vi "S7NetCom Simple Reply Decoder.vi"(11 "Live data":T1[](array[typedef])=[50, 3, 0, 0, 4, 47, 0, 2, 0, 5, 0, 0, 4, 1, 255, 4, 0, 8, 49] format="0x%02x") -> ()   [LabVIEW 2014]
doc: "____\nCopyright (c) 2019 Hampel Software Engineering (HSE), released under BSD license. More info can be found on https://dokuwiki.hampel-soft.com/code/hse/s7netcom. Original code published by Marc Christenson, Sisu Devices."
uses:
  Controls/S7NetCom_HexByte.ctl
  S7NetCom.lvclass
panel:
  out "Error":u8[](array[numeric]) format="%02x"
  out "Tab Control":enum32{"CR", "DT"}(tab)
  out "Params & Data":u8[](array[numeric]) format="%.0x"
  out "Header":u8[](array[numeric]) format="%02x"
  # "0x32\tProtocol ID"
  # "0x01 (request), 0x02 (acknowledge), 0x03 (re- sponse), \n0x07 (request user data), or 0x08 (request server control)"
  # "0x00\tReserved"
  # "0x00\tReserved"
  # "[4-5]\t\tPDU Reference (user defineable)"
  # "[6-7]\t\tParameter Length"
  # "[8-9]\t\tData Length"
  # "original message"
  # "Max AmQ (parallel jobs with ack) calling"
  # "Max AmQ (parallel jobs with ack) called"
  # "Actual PDU Length"
  # "Function code (F0 = CR, 04 = read)"
  # "no. of request items"
  # "Error Code:[1b] the return value of the operation, 0xff signals success. \nIn the Write Request message this field is always set to zero."
  # "type"
  # "size in bits(?)\n 8=1byte,16=2bytes..."
  # "<- actual data"
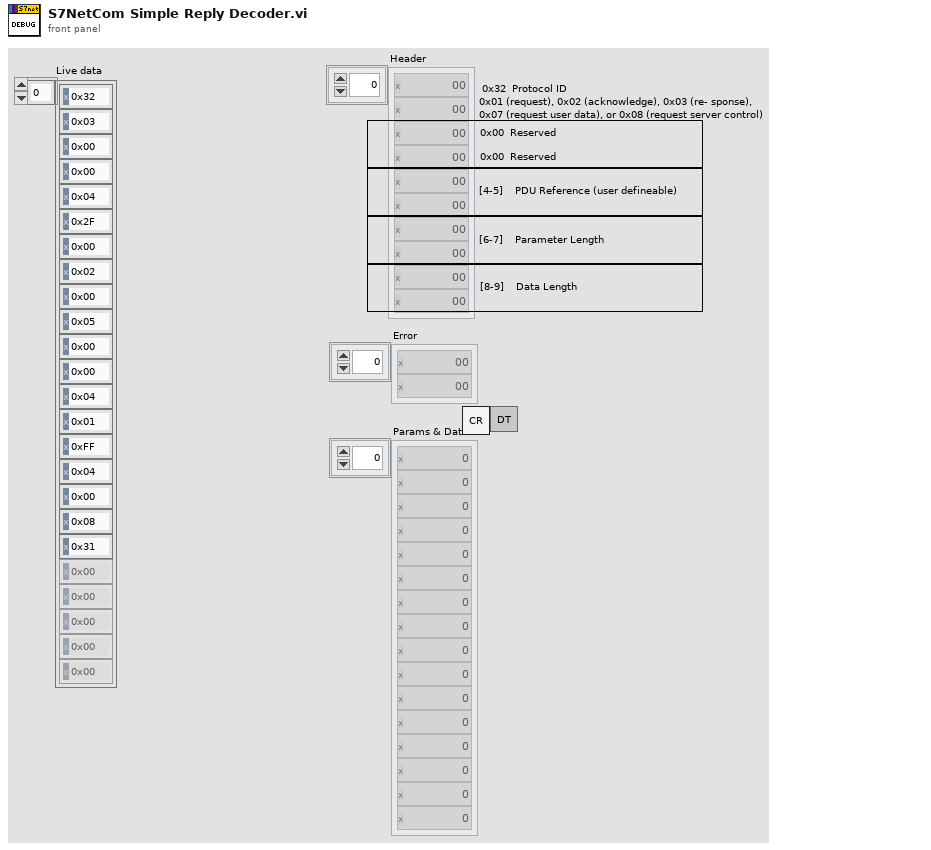
[diagram p1: front panel]
types:
  T1 = typedef "S7NetCom.lvclass/S7NetCom_HexByte.ctl" = u8
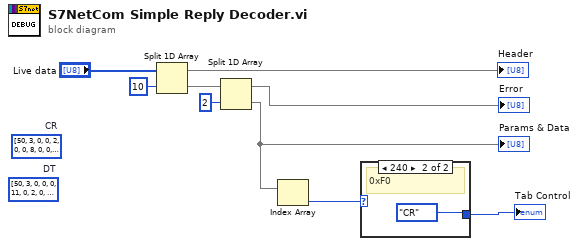
[diagram p0: block diagram]
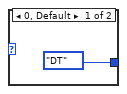
[diagram p2: hidden frame]
diagram:
  (unwired) T1[] [50, 3, 0, 0, 0, 11, 0, 2, 0, 5, 0, 0, 4, 1, 255, 4, 0, 8, 240]  # DT
  (unwired) u8[] [50, 3, 0, 0, 2, 0, 0, 8, 0, 0, 0, 0, 240, 0, 0, 1, 0, 1, 0, 240]  # CR
  n1 = Split 1D Array(array="Live data", index=10) -> (first subarray=→"Header":T1[], second subarray=w5:T1[])
  n2 = Split 1D Array(array=w5, index=2) -> (first subarray=→"Error":T1[], second subarray=w3:T1[])
  "Params & Data" <- w3
  n3 = Index Array(array=w3) -> (element=w2:T1)  [unwired: 1 in]
  n4 = case shown="240" w2 {
    tunnel: [enum32{"CR", "DT"}."DT" ("f") enum32{"CR", "DT"}."CR" ("Tab Control")] -> w1
    frame 0, Default {
    }
    frame 240 {
      # "0xF0"
    }
  }
  "Tab Control" <- w1
